vi "GetFPChildren.vi"(6 "error in":errorcluster, 9 "GObj Refnum":refnum<vi>) -> (0 "error out":errorcluster, 3 "GObj Refnum out":refnum<vi>, 4 "FP children":i32[](array[numeric]))   [LabVIEW 2014, in "Raspberry Pi Compatible Compiler for LabVIEW.lvlib" / "VI Interpreter.lvclass"]
uses:
  VI Interpreter.lvclass
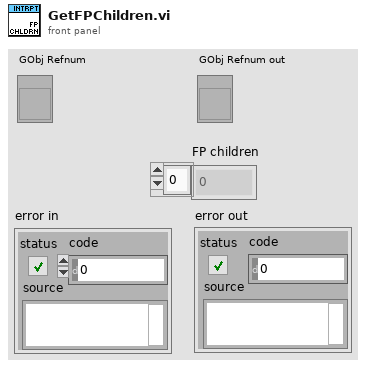
[diagram p1: front panel]
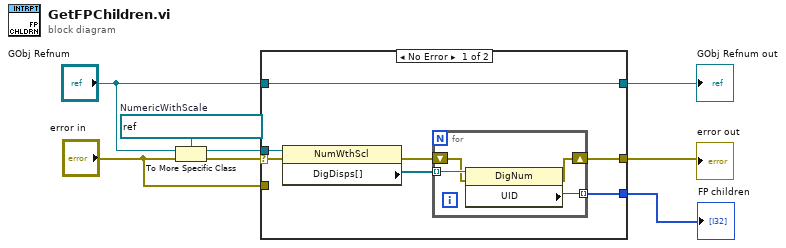
[diagram p0: block diagram]
diagram:
  w8 = refnum<vi> refnum  # NumericWithScale
  n1 = To More Specific Class(target class=w8, reference="GObj Refnum", error in="error in") -> (specific class reference=w7:refnum<vi>, error out=w6:errorcluster)
  n2 = case shown="No Error" w6 {
    selector: w6 -> [w15 _]
    tunnel: w7 -> [w14 _]
    tunnel: "GObj Refnum" -> [w9 w20]
    tunnel: [w11 _] -> w1
    tunnel: "error in" -> [_ w21]
    tunnel: [w10 w21] -> w3
    tunnel: [w9 w20] -> w2
    frame No Error {
      n3 = property class="NumWthScl"(reference=w14, error in=w15) -> (error out=w12:errorcluster, "DigDisps[]"=w13:refnum<vi>[])  [unwired: 1 out]
      n4 = for {
        tunnel: w13 -> [w19] mode=indexing
        tunnel: [w18] -> w11 mode=indexing
        shift-right: [w16] -> w10
        shift-left: w12 -> [w17]
        n5 = property class="DigNum"(reference=w19, error in=w17) -> (error out=w16:errorcluster, "UID"=w18:i32)  [unwired: 1 out]
      }
    }
    frame Error {
    }
  }
  "error out" <- w3
  "GObj Refnum out" <- w2
  "FP children" <- w1
